vi "Get Temperature Stability.vi"(8 "error in":errorcluster, 11 "TEC 1090 in":refnum<class "Meerstetter TEC.lvclass">) -> (0 "error out":errorcluster, 2 "Number":i32=93, 3 "TEC 1090 out":refnum<class "Meerstetter TEC.lvclass">)   [LabVIEW 2014, in "Meerstetter Lib.lvlib" / "Meerstetter TEC.lvclass"]
uses:
  Meerstetter TEC.lvclass
  Controls/Read Parameters.ctl
  reusable/Session APIs/Serial/Serial Session.lvclass
  Meerstetter TEC.lvclass/Meerstetter TEC.ctl
  reusable/Session APIs/Serial/Public/Asynchronous Write.vi
  reusable/Session APIs/Serial/Public/Asynchronous Read.vi
panel:
  out "substring":string
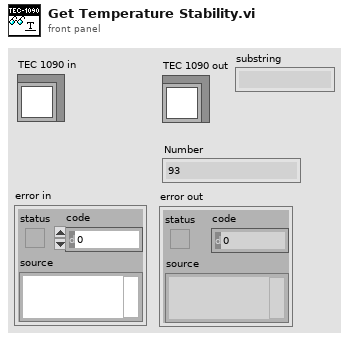
[diagram p1: front panel]
types:
  T1 = typedef "Read Parameters.ctl" = u16
  T2 = typedef "Session - Root.lvclass/Session Handle.ctl" = refnum<data-value>
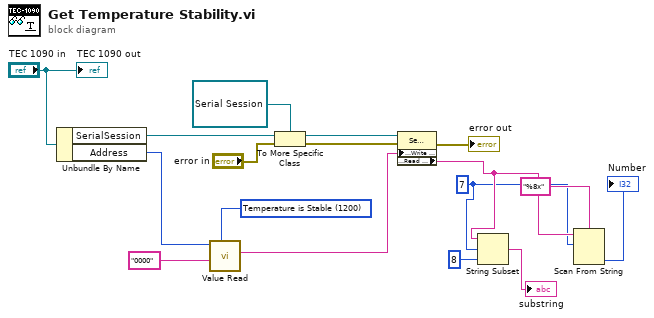
[diagram p0: block diagram]
diagram:
  w3 = 7 ("offset (0)")
  w17 = T1 1200 items=["Device Type"=100, "Hardware Version"=101, "Serial Number"=102, "Firmware Version"=103, "Device Status"=104, "Error Number"=105, "Error Instance"=106, "Error Parameter"=107, "Save Data to Flash"=108, "Flash Status"=109, "Object Temperature"=1000, "Sink Temperature"=1001, "Target Obj Temperature"=1010, "Nominal Obj Temperature"=1011, "Thermal Power Mod Current"=1012, "Actual Output Current"=1020, "Actual Output Voltage"=1021, "Relative Cooling Power"=1100, "Nominal Fan Speed"=1101, "Actual Fan Speed"=1102, "Fan PWM Level"=1103, "PID Lower Limitation"=1030, "PID Upper Limitation"=1031, "PID Control Variable"=1032, "Obj Sensor Raw ADC Val"=1040, "Sink Sensor Raw ADC Val"=1041, "Object Sensor Resistance"=1042, "Sink Sensor Resistance"=1043, "Driver Input Voltage"=1060, "10V Internal Supply"=1061, "3.3V Internal Supply"=1062, "Base Plate Temperature"=1063, "Error Number"=1070, "Error Instance"=1071, "Error Parameter"=1072, "Temperature is Stable"=1200] ("Read Values")
  n1 = Unbundle By Name("TEC 1090 in") -> ("SerialSession"=w15:T2, "Address"=w7:u8)
  n2 = call "Value Read.vi"("Read Values"=w17, "Sequence"="0000", "Address"=w7) -> ("hex integer string"=w12:string)  [unwired: 8 in]
  n3 = To More Specific Class(target class=refnum<data-value> refnum, reference=w15, error in="error in") -> (specific class reference=w13:refnum<data-value>, error out=w10:errorcluster)
  n4 = property class="Serial Session"(reference=w13, error in=w10, "Public:Write - Asynchronous"=w12) -> (error out=→"error out":errorcluster, "Public:Read - Asynchronous"=w4:string)  [unwired: 1 out]
  n5 = String Subset(string=w4, offset (0)=w3, length (rest)=8 ("length (rest)")) -> (substring=→"substring":string)
  n6 = Scan From String(format string="%8x", input string=w4, initial scan location=w3) -> (output 1=→"Number":i32)  [unwired: 2 in, 3 out]
  "TEC 1090 out" <- "TEC 1090 in"
